vi "SetFs.vi"(8 "error in (no error)":errorcluster, 9 "Fs":dbl format="%#_6pHz", 10 "Port":string(combo), 11 "reference in":refnum<class "niMmWave_Reciever.lvclass">) -> (0 "error out":errorcluster, 3 "reference out":refnum<class "niMmWave_Reciever.lvclass">)   [LabVIEW 2019, in "niMmWave_Reciever.lvclass"]
doc: "Set sampling frequency for port"
uses:
  niMmWave_Reciever.lvclass
  mmWave instrument_class/mmWave instrument.lvclass
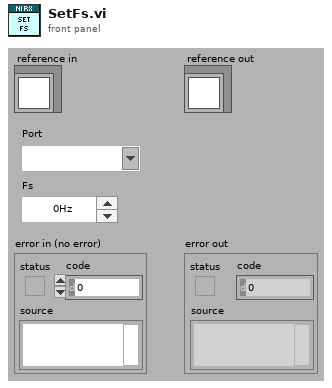
[diagram p1: front panel]
types:
  T1 = typedef "niMmWave_Reciever.lvclass/ObjectAttributesRef.ctl" = refnum<data-value>
  T2 = typedef "niMmWave_Reciever.lvclass/ObjectAttributes.ctl" = cluster{"session":T3[], "HW.RX devices":T17, "RF config":T18, "RX trigger options":T19, "RX samples":i32, "RX Fs":dbl}
  T3 = typedef "Session.ctl" = cluster{"3620 session":refnum<queue>, "tx baseband session":T4, "rx baseband session":T12, "tx gain (dB)":dbl, "rx gain (dB)":dbl, "hardware configuration":T13, "gain ranging":T15[], "pxi trigger bus information":T16}
  T4 = typedef "Tx Baseband Session.ctl" = cluster{"3610 session":T5, "7902 reference":T11}
  T5 = typedef "ni3610_and_ni3630_Driver_Lib.lvlib/Main Settings.ctl" = cluster{"VISA resource name":refnum<visa-resource-name>, "Address Space":T6, "window_offset":u32, "register_addresses":T7, "required_MM_fpga_version":cluster{"signature":u32, "hardware":u32, "current revision":u32, "oldest revision":u32}, "CPLD Oldest Compat Version ":cluster{"hardware":u32, "CPLD firmware":u32}, "MM_FPGA_image_location":string, "is_init":bool, "card_type":T8, "DacLmkConfigFileName":string, "AdcLmkConfigFileName":string, "AdcConfigFileName":string, "DacConfigFileName_RevA":string, "DacConfigFileName_RevB":string, "Mulde hardware revision":u8, "bypass DAC PLL\n":bool, "IQ Card Revision":T9, "board capability":T10}
  T6 = typedef "VISA Register Access Address Space.ctl" = u16
  T7 = typedef "ni3610_and_ni3630_Driver_Lib.lvlib/Register Adresses.ctl" = cluster{"MM based Registers":cluster{"Revision":u32, "OldestCompatRev":u32, "signature":u32, "scratch":u32, "LedControl":u32, "BoardHwRev":u32, "BoardControl":u32, "ThermalStatus":u32, "BasebandStatus":u32, "BasebandControl":u32, "BasebandAuxSetup":u32, "BasebandAuxStatus":u32, "LmkSyncOutSetup":u32, " AdcSyncOutSetup":u32, " InjSyncOutSetup":u32, " PxiTrig0OutSetup":u32, " PxiTrig1OutSetup":u32, " PxiTrig2OutSetup":u32, " PxiTrig3OutSetup":u32, " PxiTrig4OutSetup":u32, " PxiTrig5OutSetup":u32, " PxiTrig6OutSetup":u32, " PxiTrig7OutSetup":u32}, "CPLD based Registers":cluster{"SlaveSignature":u32, "SlaveRevision":u32, "SlaveOldestCompatRev":u32, "SlaveScratch":u32, "SlaveSetup":u32, "SlaveStatus":u32, "IDacReg_offset":u32, "LMKRegGrp0_offset":u32, "QDacReg_offset":u32, "BrdTempSensorVal":u32, "TempSensorPowerDown":u32, "GPIOReg_offset":u32, "IAdcReg_offset":u32, "QAdcReg_offset":u32, "LMKRegGrp1_offset":u32, "QadcTempSensorVal":u32, "IadcTempSensorVal":u32, "RevisionReg":u32, "VcxoReg":u32, "CpldStatusReg":u32, "PowerReg":u32, "VBiasEnReg":u32, "ExtRefOeReg":u32, "QdacCtrlReg":u32, "QdacStatusReg":u32, "IdacCtrlReg":u32, "IdacStatusReg":u32, "QdacJtagIn":u32, "QdacJtagOut":u32, "IdacJtagIn":u32, "IdacJtagOut":u32, "IqDcSetupReg":u32, "QadcStatusReg":u32, "IadcStatusReg":u32, "BrdSetupReg":u32, "IqDcRevisionReg":u32, "PllStatusReg":u32, "EndpointScratchReg":u32, "AdcSyncCfgReg":u32, "IqCardOpampReg":u32}, "CPLD Register Offset":u32, "MM  Register Offset":u32, " PxiTrig0OutSetup":u32}
  T8 = typedef "ni3610_and_ni3630_Driver_Lib.lvlib/Base Card Type.ctl" = enum16{"unspecified", "ADC", "DAC"}
  T9 = typedef "ni3610_and_ni3630_Driver_Lib.lvlib/IQ Card Revision.ctl" = enum16{"RevA", "RevB", "RevC", "RevD"}
  T10 = typedef "ni3610_and_ni3630_Driver_Lib.lvlib/Board Capability.ctl" = cluster{"baseband sync":enum16{"no baseband sync", "baseband sync"}}
  T11 = typedef "Blank FPGA Reference.ctl" = refnum<k20>
  T12 = typedef "Rx Baseband Session.ctl" = cluster{"3630 session":T5, "7902 reference":T11}
  T13 = typedef "Hardware Configuration.ctl" = cluster{"direction":T14, "baseband only":bool}
  T14 = typedef "Direction.ctl" = enum16{"Transceiver", "Receiver", "Transmitter"}
  T15 = typedef "Gain Ranging.ctl" = cluster{"gain ranging active scope":string, "gain ranging stream session":refnum<k20>}
  T16 = typedef "PXI Trigger Bus Info.ctl" = cluster{"chassis resource name":refnum<visa-resource-name>, "7902R (TX)":i16, "3610 (TX)":i16, "3620 (IF)":i16, "3630 (RX)":i16, "7902R (RX)":i16}
  T17 = typedef "mmWave HW Control.lvlib/HW RX resources cluster.ctl" = cluster{"HW.IF":tag, "HW.ADC":refnum<visa-resource-name>, "HW.RX FPGA":tag}
  T18 = typedef "mmWave HW Control.lvlib/HW RX RF config cluster.ctl" = cluster{"Gain":dbl, "Frequency":dbl, "mmWave adapter":string}
  T19 = typedef "TX trigger config.ctl" = cluster{"delay":dbl, "trig source":T20, "PXI src":i32, "export":T21, "PXI dest":i32}
  T20 = typedef "FPGA Utility.lvlib/FPGA driver trigger source.ctl" = enum16{"Use Tclk", "PXI_Trig", "Aurora RX trig"}
  T21 = typedef "FPGA Utility.lvlib/FPGA driver trigger destination.ctl" = enum16{"None", "Source trig", "Synced trig", "Delayed sync"}
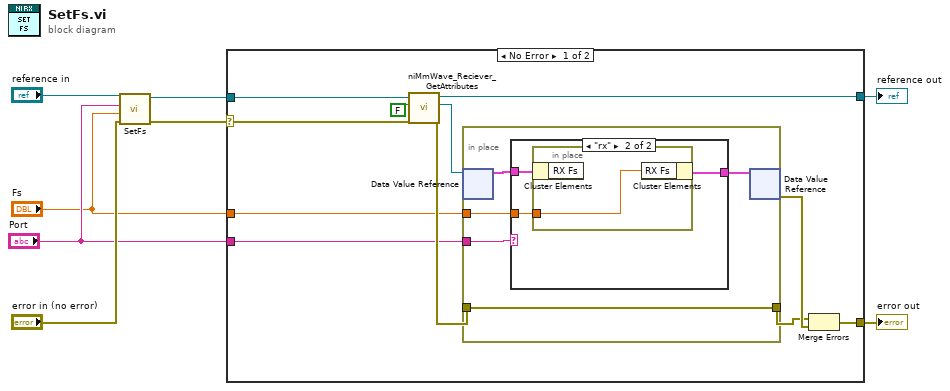
[diagram p0: block diagram]
diagram:
  n1 = call-parent "SetFs.vi"("error in (no error)"="error in (no error)", "Fs"="Fs", "Port"="Port", "reference in"="reference in") -> ("error out"=w5:errorcluster, "reference out"=w4:refnum<class "niMmWave_Reciever.lvclass">)  [unwired: 6 in]
  n2 = case shown="No Error" w5 {
    selector: w5 -> [w12 w30]
    tunnel: [w19 w30] -> w8
    tunnel: [w14 w31] -> w6
    tunnel: w4 -> [w11 w31]
    tunnel: "Port" -> [w10 _]
    tunnel: "Fs" -> [w9 _]
    frame No Error {
      n3 = call "niMmWave_Reciever_GetAttributes.vi"("error in (no error)"=w12, "return data? (T)"=FALSE, "reference in"=w11) -> ("error out"=w15:errorcluster, "attributes ref"=w13:T1, "reference out"=w14:refnum<class "niMmWave_Reciever.lvclass">)  [unwired: 5 in, 1 out]
      n4 = in-place {
        in-place-border: w15 -> [w22]
        in-place-border: [w22] -> w17
        in-place-border: w10 -> [w21]
        in-place-border: w9 -> [w20]
        n5 = in-place-dvr #1(w13) -> (w23:T2)  [unwired: 1 out]
        n6 = case shown="\"rx\"" w21 {
          tunnel: [w25 w28] -> w24
          tunnel: w23 -> [w25 w27]
          tunnel: w20 -> [_ w26]
          frame "False", Default {
          }
          frame "rx" {
            n7 = in-place {
              in-place-border: w26 -> [w29]
              n8 = in-place-cluster #2(w27) -> ()  [unwired: 1 out]
              n9 = in-place-cluster #2("RX Fs"=w29) -> (w28:T2)
            }
          }
        }
        n10 = in-place-dvr #1(w24) -> (w18:errorcluster)  [unwired: 1 out]
      }
      n11 = Merge Errors(w17, w18) -> (w19:errorcluster)
    }
    frame Error {
    }
  }
  "error out" <- w8
  "reference out" <- w6
